vi "Auto_Routine_DepositBalance.vi"(8 "error in (no error)":errorcluster) -> (0 "error out":errorcluster)   [LabVIEW 2023]
doc: "Deposites a cone on the upper node then balances\nInputs:\n--ErrorIn--\nOutputs:\n--ErrorOut--"
uses:
  Arm/ArmGamePiecePreset.ctl
  Arm/ArmPositionPreset.ctl
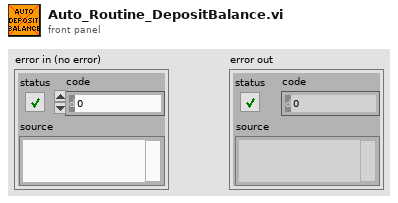
[diagram p1: front panel]
types:
  T1 = typedef "ArmGamePiecePreset.ctl" = enum16{"Cube", "Cone"}
  T2 = typedef "ArmPositionPreset.ctl" = enum16{"Upper", "Lower", "Middle", "Home", "Shelf", "Floor", "HalfFloor", "HalfHome"}
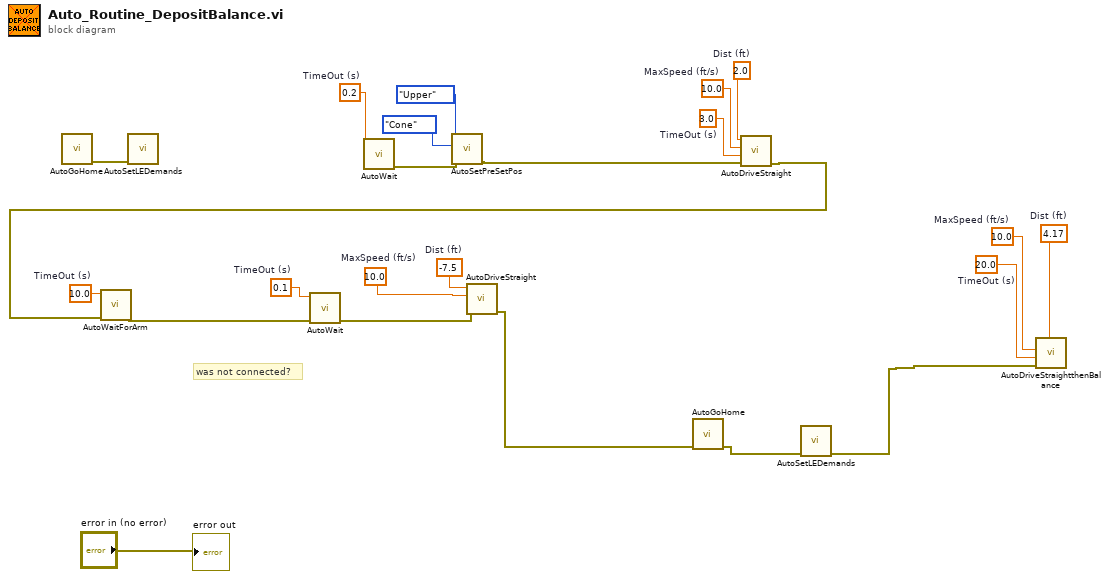
[diagram p0: block diagram]
diagram:
  w19 = 20.0  # TimeOut (s)
  w18 = 4.17  # Dist (ft)
  w17 = 10.0  # MaxSpeed (ft/s)
  w16 = 10.0  # MaxSpeed (ft/s)
  w23 = 3.0  # TimeOut (s)
  w22 = 10.0  # MaxSpeed (ft/s)
  w21 = 2.0  # Dist (ft)
  w14 = -7.5  # Dist (ft)
  w13 = 0.1  # TimeOut (s)
  w12 = 10.0  # TimeOut (s)
  w10 = 0.2  # TimeOut (s)
  # "was not connected?"
  n1 = call "AutoGoHome.vi"() -> ("error out"=w2:errorcluster)  [unwired: 11 in]
  n2 = call "AutoSetLEDemands.vi"("error in (no error)"=w2) -> ()  [unwired: 10 in, 1 out]
  n3 = call "AutoWait.vi"("TimeOut (s)"=w10) -> ("error out"=w11:errorcluster)  [unwired: 10 in]
  n4 = call "AutoSetPreSetPos.vi"("error in (no error)"=w11, "Game Piece"=ArmGamePiecePreset."Cone", "Position"=ArmPositionPreset."Upper") -> ("error out"=w5:errorcluster)  [unwired: 8 in]
  n5 = call "AutoDriveStraight.vi"("error in (no error)"=w5, "TimeOut (s)"=w23, "MaxSpeed (ft/s)"=w22, "Dist (ft)"=w21) -> ("error out"=w20:errorcluster)  [unwired: 7 in]
  n6 = call "AutoWaitForArm.vi"("error in (no error)"=w20, "TimeOut (s)"=w12) -> ("error out"=w1:errorcluster)  [unwired: 9 in]
  n7 = call "AutoWait.vi"("error in (no error)"=w1, "TimeOut (s)"=w13) -> ("error out"=w15:errorcluster)  [unwired: 9 in]
  n8 = call "AutoDriveStraight.vi"("error in (no error)"=w15, "MaxSpeed (ft/s)"=w16, "Dist (ft)"=w14) -> ("error out"=w3:errorcluster)  [unwired: 8 in]
  n9 = call "AutoGoHome.vi"("error in (no error)"=w3) -> ("error out"=w4:errorcluster)  [unwired: 10 in]
  n10 = call "AutoSetLEDemands.vi"("error in (no error)"=w4) -> ("error out"=w6:errorcluster)  [unwired: 10 in]
  n11 = call "AutoDriveStraightthenBalance.vi"("error in (no error)"=w6, "TimeOut (s)"=w19, "MaxSpeed (ft/s)"=w17, "Dist (ft)"=w18) -> ()  [unwired: 7 in, 1 out]
  "error out" <- "error in (no error)"
